vi "CRYPEAQ OurGroup.vi"(4 "Fs":dbl=48000.0, 6 "NF":dbl=2048.0, 8 "E":dbl[](array[numeric]), 9 "Fu":dbl[](array[numeric])=[21.503753670287526, 21.995027812526367, 22.49808677153995, 23.01321324469517, 23.54069671077963, 24.080833592676257, 24.63392742394026, 25.200289019371485, 25.780236649679335, 26.374096220336778, 26.982201454725374, 27.604894081673166, 28.242524027491754, 28.895449612619448, 29.564037752982106, 30.248664166183676, 30.949713582643696, 31.667579961798626, 32.40266671349049, 33.155386924665436, 33.92616359151083, 34.715429857160736, 35.523629255103735, 36.35121595842953, 37.19865503505437, 38.06642270906948, 38.95500662835802, 39.864906138632236, 40.796632564044245, 41.75070949452802, 42.72767308003404, 43.7280723318227, 44.75246943098479, 45.80144004436278, 46.87557364805095, 47.97547385865509, 49.101758772499316, 50.255061312969254, 51.4360295861875, 52.645327245221225, 53.883633863026795, 55.1516453143401, 56.45007416672793, 57.77965008102029, 59.14112022134854, 60.53524967501846, 61.962821882457085, 63.42463907747179, 64.92152273807125, 66.45431404810013, 68.02387436994864, 69.63108572860061, 71.27685130729282, 72.96209595506592, 74.68776670648897, 76.45483331385198, 78.26428879212452, 80.11714997698759, 82.014458096251, 83.95727935497855, 85.94670553464874, 87.98385460668914, 90.06987136072814, 92.20592804791596, 94.39322503968047, 96.63299150228346, 98.92648608755896, 101.27499764022106, 103.67984592213872, 106.14238235398503, 108.66399077467715, 111.2460882190335, 113.89012571408661, 116.59758909449751, 119.3699998375299, 122.2089159180549, 125.11593268406578, 128.09268375319414, 131.14084193073214, 134.26212014967754, 137.45827243332695, 140.73109488096122, 144.08242667717633, 147.5141511254243, 151.02819670634955, 154.62653816151035, 158.31119760309915, 162.0842456502813, 165.9478025927939, 169.90403958245668, 173.9551798532657, 178.10349997075375, 182.3513311113239, 186.70106037226682, 191.15513211320663, 195.71604932972951, 200.38637505995223, 205.16873382484306, 210.06581310308843, 215.0803648413393, 220.2152070006847, 225.47322514022554, 230.8573740386352, 236.37067935461374, 242.0162393271803, 247.79722651674672, 253.716889587962, 259.7785551353198, 265.9856295525604, 272.34160094691686, 278.85004109928076, 285.51460747138714, 292.33904526115157, 299.3271895073089, 306.48296724453775, 313.8103997102847, 321.31360460452737, 328.9967984037413, 336.8642987303777, 344.9205267791827, 353.1700098017141, 361.6173836504637, 370.2673953840027, 379.1249059346292, 388.1948928399923, 397.4824530402616, 406.9928057423839, 416.73129535305054, 426.70339448202407, 436.9147070175057, 447.3709712752823, 458.07806322340883, 469.04199978424884, 480.2689422157235, 491.76519957367236, 503.5372322572703, 515.591655639492, 527.9352437846665, 540.5749332552051, 553.5178270096526, 566.7711983942391, 580.3424952301918, 594.2393439990819, 608.4695541285797, 623.0411223810147, 637.9622373472125, 653.241284048125, 668.886848646851, 684.9077232736864, 701.3129109669262, 718.1116307321746, 735.3133227230385, 752.9276535460717, 770.9645216929978, 789.4340631032348, 808.3466568598475, 827.7129310221544, 847.5437685982278, 867.8503136606711, 888.6439776091183, 909.936445582935, 931.7396830277646, 954.0659424195927, 976.9277701501098, 1000.3380135772325, 1024.309828244771, 1048.8566852752717, 1073.992378940207, 1099.7310344117604, 1126.0871157005527, 1153.075433783806, 1180.7111549284552, 1209.0098092139444, 1237.9872992594592, 1267.6599091605058, 1298.0443136398683, 1329.1575874180867, 1361.0172148087065, 1393.6410995437075, 1427.047574834629, 1461.255413675032, 1496.2838393901259, 1532.1525364394283, 1568.8816614785885, 1606.4918546865524, 1645.004251364457, 1684.4404938127452, 1724.822743493209, 1766.173693482768, 1808.5165812259997, 1851.8752015935756, 1896.2739202539512, 1941.7376873658154, 1988.292051598992, 2035.9631744917108, 2084.77784515224, 2134.7634953132024, 2185.9482147470367, 2238.3607670512247, 2292.0306058121905, 2346.987891156945, 2403.2635067017727, 2460.8890769074746, 2519.896984850965, 2580.3203904231455, 2642.193248963338, 2705.550330340712, 2770.427238493444, 2836.8604314366003, 2904.887241749946, 2974.545897557262, 3045.8755440088744, 3118.9162652795458, 3193.709107094056, 3270.296099793104, 3348.720281952559, 3429.0257245692496, 3511.257555827002, 3595.4619864566853, 3681.68633570466, 3769.9790579241567, 3860.38976980449, 3952.9692782535367, 4047.7696089489996, 4144.844035574564, 4244.24710975746, 4346.034691724041, 4450.263981690873, 4556.993552008765, 4666.283380077891, 4778.194882052486, 4892.790947354097, 5010.135974012663, 5130.29590485548, 5253.338264564175, 5379.332197620682, 5508.348507163433, 5640.459694775663, 5775.740001228165, 5914.265448199384, 6056.113880996325, 6201.36501230021, 6350.100466961611, 6502.403827870036, 6658.360682923942, 6818.0586731273515, 6981.587541840409, 7149.039185211186, 7320.507703817386, 7496.08945554674, 7675.883109746058, 7859.989702669079, 8048.512694254444, 8241.558026265742, 8439.234181826203, 8641.652246381524, 8848.925970125041, 9061.17183192046, 9278.509104757919, 9501.059922780241, 9728.94934991705, 9962.30545016528, 10201.2593595556, 10445.945359845213, 10696.50095397833, 18000.0765] format="%#.6g", 10 "Fc":dbl[](array[numeric])=[20.479765400273834, 20.971039542512674, 21.474098501526257, 21.989224974681477, 22.516708440765942, 23.056845322662564, 23.609939153926568, 24.176300749357793, 24.756248379665642, 25.350107950323086, 25.958213184711685, 26.580905811659473, 27.21853575747806, 27.871461342605755, 28.540049482968413, 29.224675896169984, 29.925725312630004, 30.643591691784934, 31.378678443476797, 32.13139865465174, 32.90217532149714, 33.69144158714705, 34.49964098509004, 35.32722768841584, 36.17466676504068, 37.04243443905579, 37.93101835834433, 38.84091786861855, 39.77264429403055, 40.72672122451433, 41.70368481002035, 42.70408406180901, 43.7284811609711, 44.77745177434909, 45.851585378037264, 46.951485588641404, 48.07777050248563, 49.23107304295556, 50.41204131617381, 51.621338975207536, 52.8596455930131, 54.127657044326405, 55.42608589671424, 56.7556618110066, 58.11713195133485, 59.511261405004774, 60.938833612443396, 62.40065080745809, 63.89753446805755, 65.43032577808644, 66.99988609993495, 68.60709745858692, 70.25286303727913, 71.93810768505223, 73.66377843647528, 75.43084504383829, 77.24030052211083, 79.0931617069739, 80.99046982623732, 82.93329108496486, 84.92271726463505, 86.95986633667545, 89.04588309071445, 91.18193977790227, 93.36923676966678, 95.60900323226977, 97.90249781754527, 100.25100937020737, 102.65585765212504, 105.11839408397134, 107.64000250466346, 110.2220999490198, 112.86613744407292, 115.57360082448382, 118.34601156751621, 121.18492764804121, 124.0919444140521, 127.06869548318045, 130.11685366071845, 133.23813187966385, 136.43428416331327, 139.70710661094753, 143.05843840716264, 146.4901628554106, 150.00420843633586, 153.60254989149666, 157.28720933308546, 161.06025738026761, 164.9238143227802, 168.880051312443, 172.931191583252, 177.07951170074006, 181.3273428413102, 185.67707210225313, 190.13114384319294, 194.69206105971583, 199.36238678993854, 204.14474555482937, 209.04182483307474, 214.05637657132561, 219.191218730671, 224.44923687021185, 229.8333857686215, 235.34669108460005, 240.9922510571666, 246.77323824673303, 252.6929013179483, 258.75456686530606, 264.9616412825467, 271.31761267690314, 277.82605282926704, 284.4906192013734, 291.31505699113785, 298.3032012372952, 305.45897897452403, 312.78641144027097, 320.28961633451365, 327.9728101337276, 335.840310460364, 343.896538509169, 352.1460215317004, 360.59339538045003, 369.243407113989, 378.1009176646155, 387.1709045699786, 396.4584647702479, 405.9688174723702, 415.7073070830368, 425.67940621201035, 435.890718747492, 446.34698300526856, 457.0540749533951, 468.0180115142351, 479.24495394570977, 490.74121130365864, 502.5132439872566, 514.5676673694784, 526.9112555146528, 539.5509449851914, 552.4938387396389, 565.7472101242255, 579.3185069601782, 593.2153557290683, 607.445565858566, 622.017134111001, 636.9382490771989, 652.2172957781113, 667.8628603768374, 683.8837350036728, 700.2889226969126, 717.0876424621609, 734.2893344530248, 751.9036652760581, 769.9405334229841, 788.4100748332212, 807.3226685898338, 826.6889427521407, 846.5197803282141, 866.8263253906574, 887.6199893391047, 908.9124573129213, 930.715694757751, 953.041954149579, 975.9037818800962, 999.3140253072188, 1023.2858399747574, 1047.832697005258, 1072.9683906701932, 1098.7070461417468, 1125.063127430539, 1152.0514455137923, 1179.6871666584416, 1207.9858209439308, 1236.9633109894455, 1266.6359208904921, 1297.0203253698546, 1328.133599148073, 1359.9932265386929, 1392.6171112736938, 1426.0235865646152, 1460.2314254050184, 1495.2598511201122, 1531.1285481694147, 1567.8576732085749, 1605.4678664165388, 1643.9802630944434, 1683.4165055427316, 1723.7987552231953, 1765.1497052127543, 1807.492592955986, 1850.851213323562, 1895.2499319839376, 1940.7136990958018, 1987.2680633289783, 2034.9391862216971, 2083.753856882226, 2133.7395070431885, 2184.924226477023, 2237.336778781211, 2291.0066175421766, 2345.963902886931, 2402.239518431759, 2459.8650886374608, 2518.872996580951, 2579.2964021531316, 2641.1692606933243, 2704.5263420706983, 2769.40325022343, 2835.8364431665864, 2903.863253479932, 2973.521909287248, 3044.8515557388605, 3117.892277009532, 3192.685118824042, 3269.27211152309, 3347.6962936825453, 3428.0017362992357, 3510.233567556988, 3594.4379981866714, 3680.662347434646, 3768.955069654143, 3859.365781534476, 3951.945289983523, 4046.7456206789857, 4143.820047304551, 4243.223121487446, 4345.010703454028, 4449.23999342086, 4555.969563738751, 4665.259391807877, 4777.170893782472, 4891.766959084083, 5009.111985742649, 5129.271916585467, 5252.314276294162, 5378.308209350668, 5507.32451889342, 5639.435706505649, 5774.716012958152, 5913.241459929371, 6055.0898927263115, 6200.341024030196, 6349.076478691598, 6501.379839600023, 6657.336694653928, 6817.034684857338, 6980.563553570396, 7148.015196941173, 7319.483715547372, 7495.065467276727, 7674.8591214760445, 7858.965714399065, 8047.48870598443, 8240.534037995729, 8438.21019355619, 8640.62825811151, 8847.901981855028, 9060.147843650446, 9277.485116487906, 9500.035934510228, 9727.925361647036, 9961.281461895267, 10200.235371285587, 10444.9213715752, 10695.476965708316, 10952.042955086945], 11 "Fl":dbl[](array[numeric])=[20.0, 21.503753670287526, 21.995027812526367, 22.49808677153995, 23.01321324469517, 23.54069671077963, 24.080833592676257, 24.63392742394026, 25.200289019371485, 25.780236649679335, 26.374096220336778, 26.982201454725374, 27.604894081673166, 28.242524027491754, 28.895449612619448, 29.564037752982106, 30.248664166183676, 30.949713582643696, 31.667579961798626, 32.40266671349049, 33.155386924665436, 33.92616359151083, 34.715429857160736, 35.523629255103735, 36.35121595842953, 37.19865503505437, 38.06642270906948, 38.95500662835802, 39.864906138632236, 40.796632564044245, 41.75070949452802, 42.72767308003404, 43.7280723318227, 44.75246943098479, 45.80144004436278, 46.87557364805095, 47.97547385865509, 49.101758772499316, 50.255061312969254, 51.4360295861875, 52.645327245221225, 53.883633863026795, 55.1516453143401, 56.45007416672793, 57.77965008102029, 59.14112022134854, 60.53524967501846, 61.962821882457085, 63.42463907747179, 64.92152273807125, 66.45431404810013, 68.02387436994864, 69.63108572860061, 71.27685130729282, 72.96209595506592, 74.68776670648897, 76.45483331385198, 78.26428879212452, 80.11714997698759, 82.014458096251, 83.95727935497855, 85.94670553464874, 87.98385460668914, 90.06987136072814, 92.20592804791596, 94.39322503968047, 96.63299150228346, 98.92648608755896, 101.27499764022106, 103.67984592213872, 106.14238235398503, 108.66399077467715, 111.2460882190335, 113.89012571408661, 116.59758909449751, 119.3699998375299, 122.2089159180549, 125.11593268406578, 128.09268375319414, 131.14084193073214, 134.26212014967754, 137.45827243332695, 140.73109488096122, 144.08242667717633, 147.5141511254243, 151.02819670634955, 154.62653816151035, 158.31119760309915, 162.0842456502813, 165.9478025927939, 169.90403958245668, 173.9551798532657, 178.10349997075375, 182.3513311113239, 186.70106037226682, 191.15513211320663, 195.71604932972951, 200.38637505995223, 205.16873382484306, 210.06581310308843, 215.0803648413393, 220.2152070006847, 225.47322514022554, 230.8573740386352, 236.37067935461374, 242.0162393271803, 247.79722651674672, 253.716889587962, 259.7785551353198, 265.9856295525604, 272.34160094691686, 278.85004109928076, 285.51460747138714, 292.33904526115157, 299.3271895073089, 306.48296724453775, 313.8103997102847, 321.31360460452737, 328.9967984037413, 336.8642987303777, 344.9205267791827, 353.1700098017141, 361.6173836504637, 370.2673953840027, 379.1249059346292, 388.1948928399923, 397.4824530402616, 406.9928057423839, 416.73129535305054, 426.70339448202407, 436.9147070175057, 447.3709712752823, 458.07806322340883, 469.04199978424884, 480.2689422157235, 491.76519957367236, 503.5372322572703, 515.591655639492, 527.9352437846665, 540.5749332552051, 553.5178270096526, 566.7711983942391, 580.3424952301918, 594.2393439990819, 608.4695541285797, 623.0411223810147, 637.9622373472125, 653.241284048125, 668.886848646851, 684.9077232736864, 701.3129109669262, 718.1116307321746, 735.3133227230385, 752.9276535460717, 770.9645216929978, 789.4340631032348, 808.3466568598475, 827.7129310221544, 847.5437685982278, 867.8503136606711, 888.6439776091183, 909.936445582935, 931.7396830277646, 954.0659424195927, 976.9277701501098, 1000.3380135772325, 1024.309828244771, 1048.8566852752717, 1073.992378940207, 1099.7310344117604, 1126.0871157005527, 1153.075433783806, 1180.7111549284552, 1209.0098092139444, 1237.9872992594592, 1267.6599091605058, 1298.0443136398683, 1329.1575874180867, 1361.0172148087065, 1393.6410995437075, 1427.047574834629, 1461.255413675032, 1496.2838393901259, 1532.1525364394283, 1568.8816614785885, 1606.4918546865524, 1645.004251364457, 1684.4404938127452, 1724.822743493209, 1766.173693482768, 1808.5165812259997, 1851.8752015935756, 1896.2739202539512, 1941.7376873658154, 1988.292051598992, 2035.9631744917108, 2084.77784515224, 2134.7634953132024, 2185.9482147470367, 2238.3607670512247, 2292.0306058121905, 2346.987891156945, 2403.2635067017727, 2460.8890769074746, 2519.896984850965, 2580.3203904231455, 2642.193248963338, 2705.550330340712, 2770.427238493444, 2836.8604314366003, 2904.887241749946, 2974.545897557262, 3045.8755440088744, 3118.9162652795458, 3193.709107094056, 3270.296099793104, 3348.720281952559, 3429.0257245692496, 3511.257555827002, 3595.4619864566853, 3681.68633570466, 3769.9790579241567, 3860.38976980449, 3952.9692782535367, 4047.7696089489996, 4144.844035574564, 4244.24710975746, 4346.034691724041, 4450.263981690873, 4556.993552008765, 4666.283380077891, 4778.194882052486, 4892.790947354097, 5010.135974012663, 5130.29590485548, 5253.338264564175, 5379.332197620682, 5508.348507163433, 5640.459694775663, 5775.740001228165, 5914.265448199384, 6056.113880996325, 6201.36501230021, 6350.100466961611, 6502.403827870036, 6658.360682923942, 6818.0586731273515, 6981.587541840409, 7149.039185211186, 7320.507703817386, 7496.08945554674, 7675.883109746058, 7859.989702669079, 8048.512694254444, 8241.558026265742, 8439.234181826203, 8641.652246381524, 8848.925970125041, 9061.17183192046, 9278.509104757919, 9501.059922780241, 9728.94934991705, 9962.30545016528, 10201.2593595556, 10445.945359845213, 10696.50095397833] format="%#.6g") -> (3 "Grouped E":dbl[](array[numeric]))   [LabVIEW 2013]
uses:
  <vilib>/Analysis/baseanly.llb/Mean (DBL).vi
  <vilib>/Analysis/NI_AALBase.lvlib
panel:
  out "P[noise] 6":cluster{"Fc":dbl[], dbl[]}(graph)
  out "max value":i32
  out "Waveform Graph":i32[](graph)
  out "df":dbl
  out "fu index":i32[](array[numeric])
  out "fl index":i32[](array[numeric])
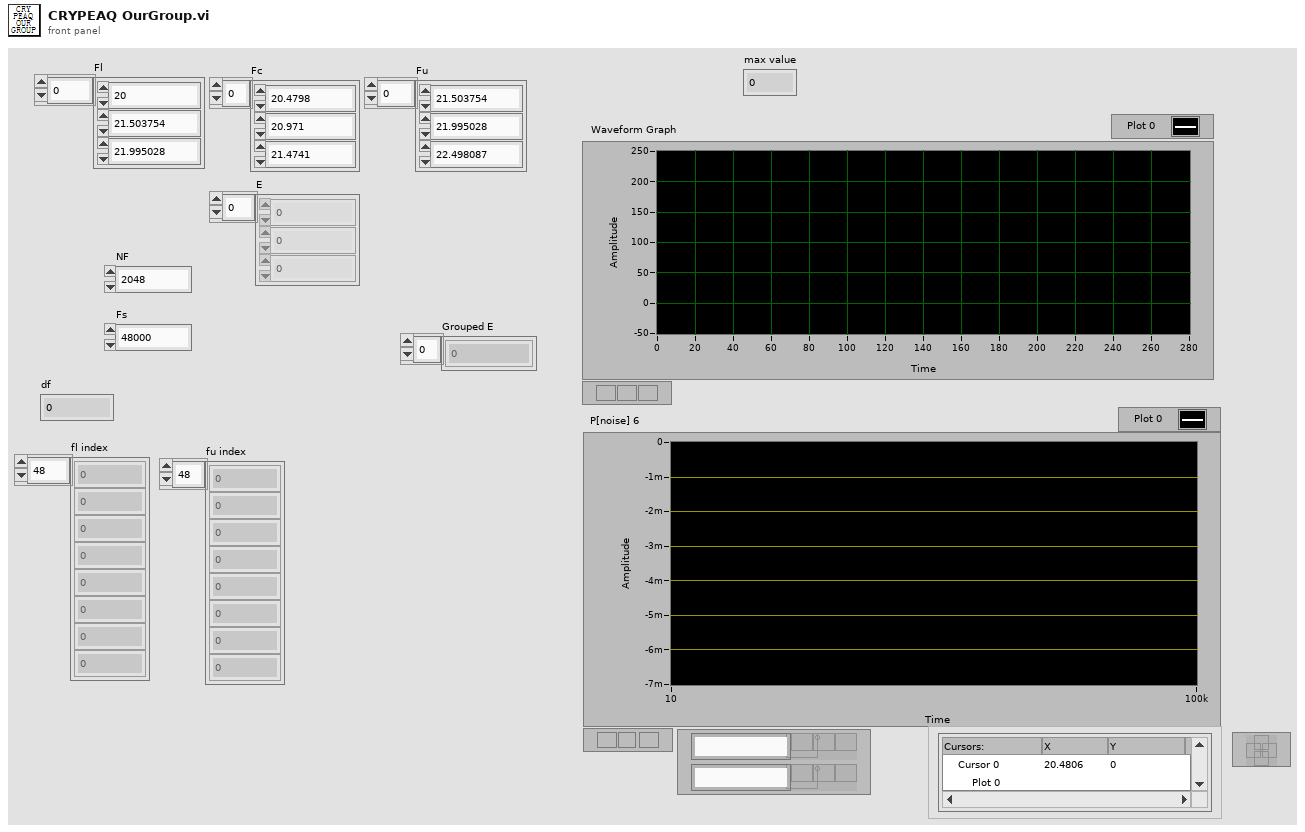
[diagram p1: front panel]
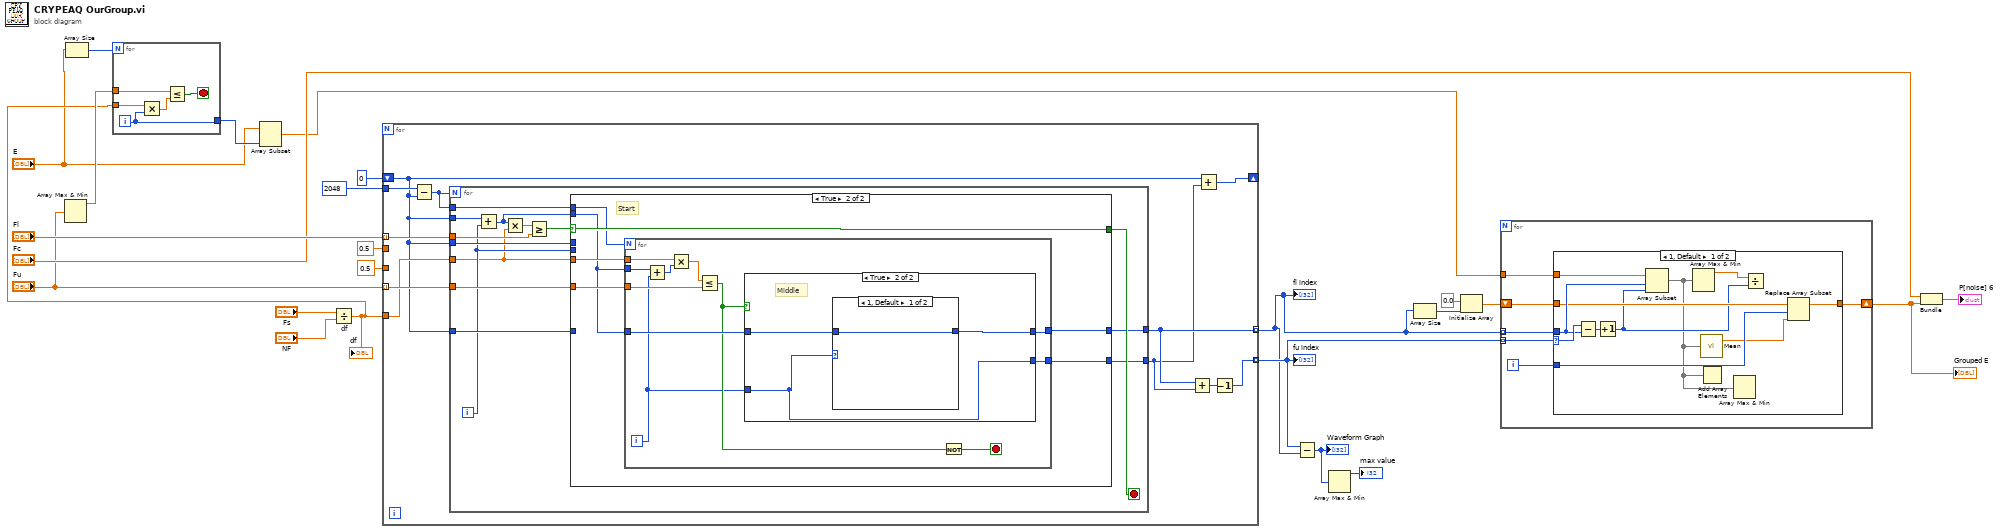
[diagram p0: block diagram]
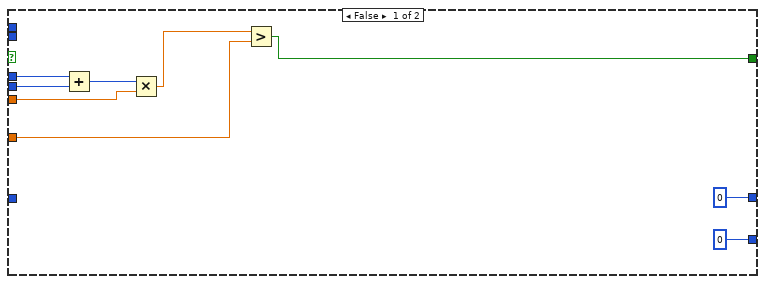
[diagram p3: hidden frame]
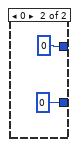
[diagram p5: hidden frame]
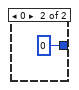
[diagram p6: hidden frame]
diagram:
  n1 = Array Max & Min(array="Fu") -> (max value=w6:dbl)  [unwired: 3 out]
  n2 = Array Size(array="E") -> (size(s)=w1:i32)
  n3 = Divide "df"(x="Fs", y="NF") -> (x/y=w5:dbl)
  "df" <- w5
  n4 = for {
    N: w1 -> [_]
    tunnel: w6 -> [w28]
    tunnel: w5 -> [w29]
    tunnel: [w25] -> w4
    i -> [w25]
    stop <- w26 stop-if-true
    n5 = Multiply(x=w29, y=w25) -> (x*y=w27:dbl)
    n6 = Less Or Equal?(x=w28, y=w27) -> (x <= y?=w26:bool)
  }
  n7 = Array Subset(array="E", length=w4) -> (w3:dbl[])  [unwired: 1 in]
  n8 = for {
    tunnel: "Fl" -> [w40] mode=indexing
    tunnel: "Fu" -> [w39] mode=indexing
    tunnel: w5 -> [w32]
    shift-right: [w37] -> _
    shift-left: 0 ("index") -> [w31]
    tunnel: 0.5 -> [_]
    tunnel: 2048 ("size(s)") -> [w38]
    tunnel: 0.5 -> [_]
    tunnel: [w36] -> w15 mode=indexing
    tunnel: [w34] -> w16 mode=indexing
    n9 = Subtract(x=w38, y=w31) -> (x-y=w30:i32)
    n10 = for {
      N: w30 -> [_]
      tunnel: w40 -> [w54]
      tunnel: w39 -> [w51]
      tunnel: w31 -> [w53]
      tunnel: [w49] -> w33
      tunnel: [w48] -> w36
      tunnel: w32 -> [w42]
      tunnel: w31 -> [w47]
      tunnel: w31 -> [w46]
      tunnel: w30 -> [w43]
      i -> [w45]
      stop <- w52 stop-if-true
      n11 = Add(x=w46, y=w45) -> (x+y=w41:i32)
      n12 = Multiply(x=w41, y=w42) -> (x*y=w44:dbl)
      n13 = Greater Or Equal?(x=w44, y=w54) -> (x >= y?=w50:bool)
      n14 = case shown="True" w50 {
        selector: w50 -> [_ w70]
        tunnel: w53 -> [_ _]
        tunnel: [w61 w70] -> w52
        tunnel: [0 w68] -> w48
        tunnel: w51 -> [w62 w69]
        tunnel: [0 w67] -> w49
        tunnel: w42 -> [w59 w66]
        tunnel: w45 -> [w58 _]
        tunnel: w47 -> [w57 _]
        tunnel: w43 -> [_ w65]
        tunnel: w41 -> [_ w64]
        frame False {
          n15 = Add(x=w57, y=w58) -> (x+y=w56:i32)
          n16 = Multiply(x=w56, y=w59) -> (x*y=w55:dbl)
          n17 = Greater?(x=w55, y=w62) -> (0:w61:bool)
        }
        frame True {
          # "Start"
          n18 = for {
            N: w65 -> [_]
            tunnel: w69 -> [w81]
            tunnel: [w80] -> w68
            tunnel: w64 -> [w79]
            tunnel: [w78] -> w67
            tunnel: w66 -> [w75]
            tunnel: w64 -> [w73]
            i -> [w72]
            stop <- w76 stop-if-true
            n19 = Add(x=w73, y=w72) -> (x+y=w74:i32)
            n20 = Multiply(x=w75, y=w74) -> (x*y=w71:dbl)
            n21 = Less Or Equal?(x=w71, y=w81) -> (x <= y?=w77:bool)
            n22 = case shown="True" w77 {
              tunnel: w72 -> [w85 w90]
              tunnel: [w83 w92] -> w80
              tunnel: w79 -> [w84 w91]
              tunnel: [w82 w90] -> w78
              frame False {
                # "End"
                n23 = case shown="1, Default" w85 {
                  selector: w85 -> [w86 _]
                  tunnel: [w87 0] -> w83
                  tunnel: w84 -> [w87 _]
                  tunnel: [w86 0] -> w82
                  frame 1, Default {
                  }
                  frame 0 {
                  }
                }
              }
              frame True {
                # "Middle"
                n24 = case shown="1, Default" w90 {
                  tunnel: [w93 0] -> w92
                  tunnel: w91 -> [w93 _]
                  frame 1, Default {
                  }
                  frame 0 {
                  }
                }
              }
            }
            n25 = Not(x=w77) -> (.not. x?=w76:bool)
          }
        }
      }
    }
    n26 = Add(x=w36, y=w33) -> (x+y=w35:i32)
    n27 = Add(x=w31, y=w33) -> (x+y=w37:i32)
    n28 = Decrement(x=w35) -> (x-1=w34:i32)
  }
  "fl index" <- w15
  "fu index" <- w16
  n29 = Subtract(x=w16, y=w15) -> (x-y=w18:i32[])
  "Waveform Graph" <- w18
  n30 = Array Max & Min(array=w18) -> (max value=→"max value":i32)  [unwired: 3 out]
  n31 = Array Size(array=w15) -> (size(s)=w14:i32)
  n32 = Initialize Array(0.0 ("element"), w14) -> (w12:dbl[])
  n33 = for {
    tunnel: w3 -> [w99]
    tunnel: w15 -> [w97] mode=indexing
    tunnel: w16 -> [w100] mode=indexing
    shift-right: [w95] -> w11
    shift-left: w12 -> [w98]
    i -> [w96]
    n34 = case shown="1, Default" w100 {
      selector: w100 -> [w110 _]
      tunnel: w99 -> [w111 _]
      tunnel: w98 -> [w107 w112]
      tunnel: w97 -> [w109 _]
      tunnel: w96 -> [w106 _]
      tunnel: [w105 w112] -> w95
      frame 1, Default {
        n35 = Subtract(x=w110, y=w109) -> (x-y=w108:i32)
        n36 = Increment(x=w108) -> (x+1=w103:i32)
        n37 = Array Subset(array=w111, index=w109, length=w103) -> (w102:dbl[])
        n38 = Array Max & Min(array=w102) -> (max value=w104:dbl)  [unwired: 3 out]
        n39 = call-poly <vilib>:"Mean.vi"("X"=w102) -> ("mean"=w101:dbl)  [unwired: 1 out]
        n40 = Add Array Elements(numeric array=w102) -> ()  [unwired: 1 out]
        n41 = Array Max & Min(array=w102) -> ()  [unwired: 4 out]
        n42 = Divide(x=w104, y=w103) -> ()  [unwired: 1 out]
        n43 = Replace Array Subset(array=w107, new element=w101, index=w106) -> (w105:dbl[])
      }
      frame ..0 {
      }
    }
  }
  "Grouped E" <- w11
  n44 = Bundle("Fc"="Fc", w11) -> (→"P[noise] 6":cluster{"Fc":dbl[], dbl[]})  [unwired: 1 in]
